vi "KL_divergance.vi"(10 "Centroid":dbl[](array[numeric]), 11 "Independent\nVariable (Zi)":dbl[](array[numeric])) -> (3 "Euclidean\nDistance":dbl)   [LabVIEW 2014]
uses:
  <vilib>/Analysis/NI_AALPro.lvlib
panel:
  out "Histogram Graph 4":T1(graph)
  out "Histogram Graph 3":T1(graph)
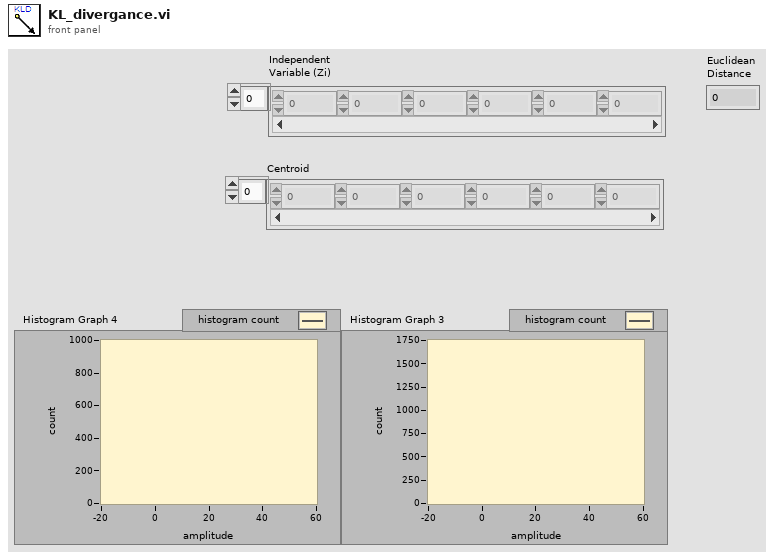
[diagram p1: front panel]
types:
  T1 = cluster{"X Values":dbl[], "Histogram: h(x)":i32[]}
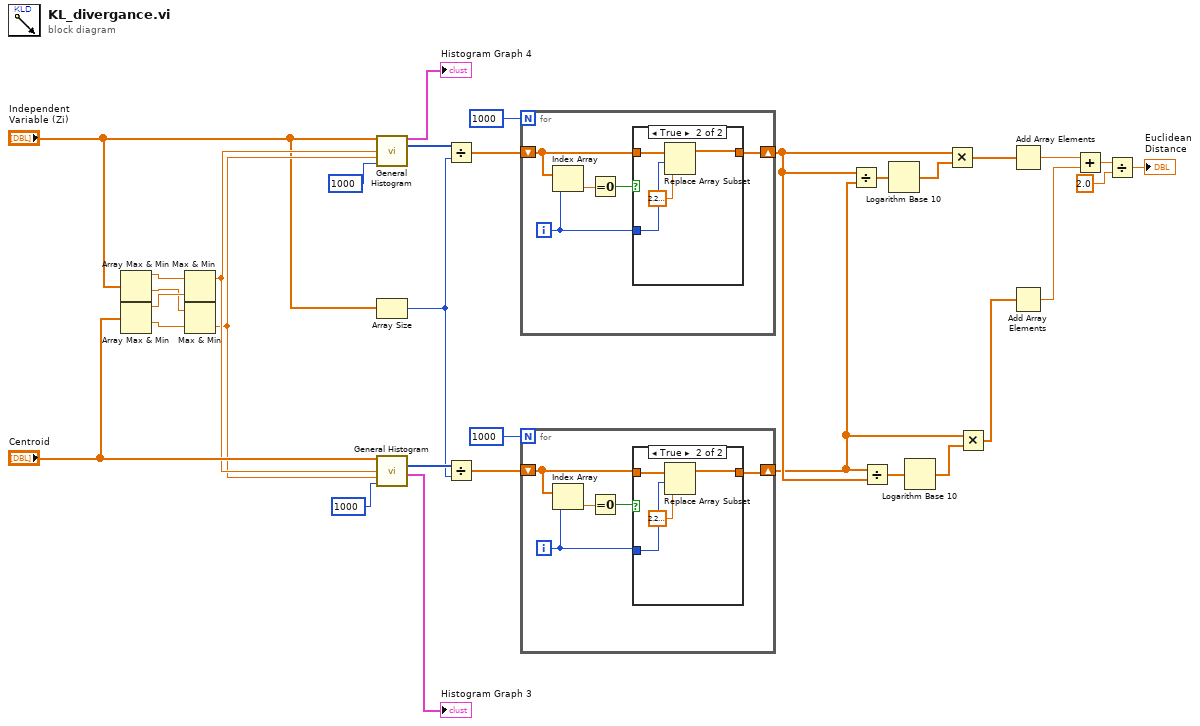
[diagram p0: block diagram]
diagram:
  n1 = Array Max & Min(array="Independent\nVariable (Zi)") -> (max value=w24:dbl, min value=w22:dbl)  [unwired: 2 out]
  n2 = Array Max & Min(array="Centroid") -> (max value=w23:dbl, min value=w21:dbl)  [unwired: 2 out]
  n3 = Max & Min(x=w24, y=w23) -> (max(x,y)=w20:dbl)  [unwired: 1 out]
  n4 = Max & Min(x=w22, y=w21) -> (min(x,y)=w19:dbl)  [unwired: 1 out]
  n5 = call <vilib>:"General Histogram.vi"("X"="Independent\nVariable (Zi)", "max"=w20, "min"=w19, "# bins"=1000) -> ("Histogram Graph"=→"Histogram Graph 4":T1, "Histogram"=w11:i32[])  [unwired: 7 in, 3 out]
  n6 = Array Size(array="Independent\nVariable (Zi)") -> (size(s)=w12:i32)
  n7 = call <vilib>:"General Histogram.vi"("X"="Centroid", "max"=w20, "min"=w19, "# bins"=1000) -> ("Histogram Graph"=→"Histogram Graph 3":T1, "Histogram"=w13:i32[])  [unwired: 7 in, 3 out]
  n8 = Divide(x=w11, y=w12) -> (x/y=w7:dbl[])
  n9 = Divide(x=w13, y=w12) -> (x/y=w9:dbl[])
  n10 = for {
    N: 1000 -> [_]
    shift-right: [w34] -> w4
    shift-left: w7 -> [w35]
    i -> [w33]
    n11 = Index Array(array=w35, index=w33) -> (element=w37:dbl)
    n12 = Equal To 0?(x=w37) -> (x = 0?=w36:bool)
    n13 = case shown="True" w36 {
      tunnel: w35 -> [w38 w42]
      tunnel: [w38 w41] -> w34
      tunnel: w33 -> [_ w40]
      frame False {
      }
      frame True {
        n14 = Replace Array Subset(array=w42, new element=2.220446049250313e-16, index=w40) -> (w41:dbl[])
      }
    }
  }
  n15 = for {
    N: 1000 -> [_]
    shift-right: [w46] -> w2
    shift-left: w9 -> [w44]
    i -> [w43]
    n16 = Index Array(array=w44, index=w43) -> (element=w47:dbl)
    n17 = Equal To 0?(x=w47) -> (x = 0?=w45:bool)
    n18 = case shown="True" w45 {
      tunnel: w44 -> [w48 w52]
      tunnel: [w48 w51] -> w46
      tunnel: w43 -> [_ w50]
      frame False {
      }
      frame True {
        n19 = Replace Array Subset(array=w52, new element=2.220446049250313e-16, index=w50) -> (w51:dbl[])
      }
    }
  }
  n20 = Divide(x=w4, y=w2) -> (x/y=w6:dbl[])
  n21 = Divide(x=w2, y=w4) -> (x/y=w3:dbl[])
  n22 = Logarithm Base 10(1:w6) -> (0:w32:dbl[])
  n23 = Logarithm Base 10(1:w3) -> (0:w31:dbl[])
  n24 = Multiply(x=w4, y=w32) -> (x*y=w5:dbl[])
  n25 = Multiply(x=w2, y=w31) -> (x*y=w1:dbl[])
  n26 = Add Array Elements(numeric array=w5) -> (sum=w30:dbl)
  n27 = Add Array Elements(numeric array=w1) -> (sum=w29:dbl)
  n28 = Add(x=w30, y=w29) -> (x+y=w28:dbl)
  n29 = Divide(x=w28, y=2.0) -> (x/y=→"Euclidean\nDistance":dbl)
